vi "getDetails.vi"(8 "error in (no error)":errorcluster, 9 "S/N":string, 11 "reference in":refnum<class "Notification Controller.lvclass">) -> (0 "error out":errorcluster, 2 "details":T2, 3 "reference out":refnum<class "Notification Controller.lvclass">)   [LabVIEW 2014, in "Notification Controller.lvclass"]
uses:
  Notification Controller.lvclass
  Devices Controller_llb/deviceType.ctl
  APP/itemsNotification_class/itemsNotification.lvclass
  Devices Controller_llb/Devices Controller.lvclass
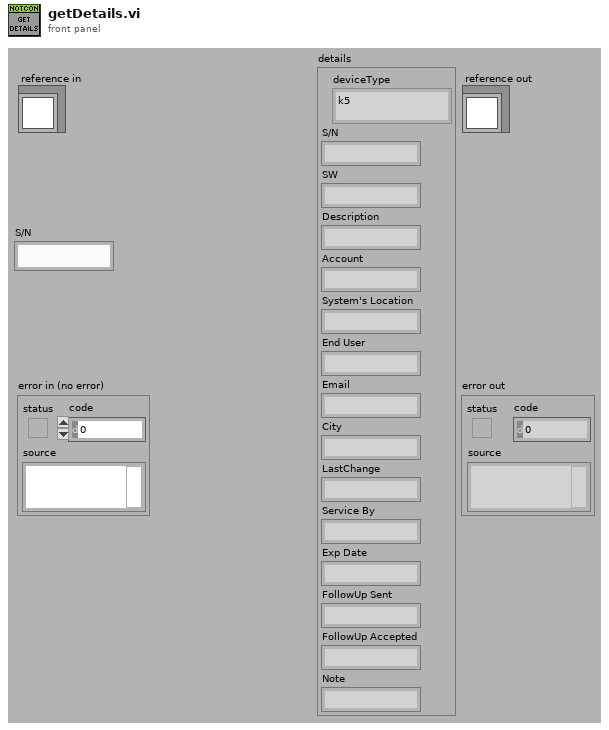
[diagram p1: front panel]
types:
  T1 = typedef "Devices Controller.lvclass/deviceType.ctl" = enum16{"k5", "k4b2", "fitmate", "cpet", "rmr", "bodyBoxPft", "bp", "pp"}
  T2 = cluster{"deviceType":T1, "S/N":string, "SW":string, "Description":string, "Account":string, "System's Location":string, "End User":string, "Email":string, "City":string, "LastChange":string, "Service By":string, "Exp Date":string, "FollowUp Sent":string, "FollowUp Accepted":string, "Note":string}
  T3 = typedef "Notification Controller.lvclass/ObjectAttributesRef.ctl" = refnum<data-value>
  T4 = typedef "Notification Controller.lvclass/ObjectAttributes.ctl" = cluster{"MyAttribute":dbl, "items_data":string[][][], "items_notification_refs":refnum<class "itemsNotification.lvclass">[], "notifications_data_items":string[][], "items_nots?":bool, "devices_controller_ref":refnum<class "Devices Controller.lvclass">, "onlineUpdate":timestamp, "notController?":bool, "tracking_notification_ref":refnum<class "trackingNotification.lvclass">, "notifications_data_tracking":string[][], "tracking_parts_data":string[][], "tracking_nots?":bool, "index_tracking_not":i32[], "file_controller_ref":refnum<class "File Controller.lvclass">}
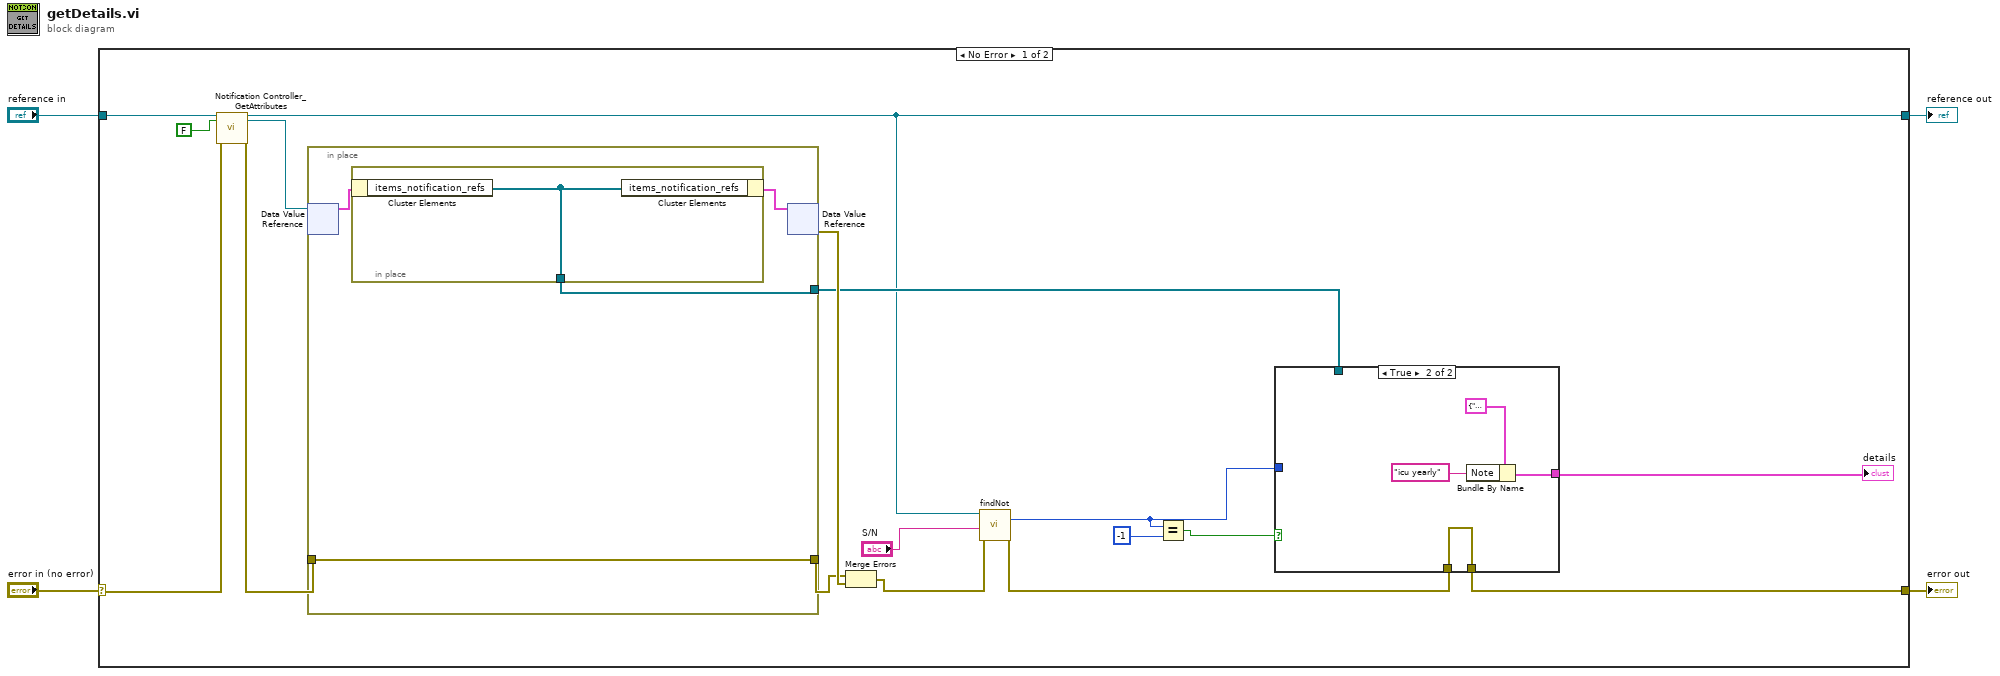
[diagram p0: block diagram]
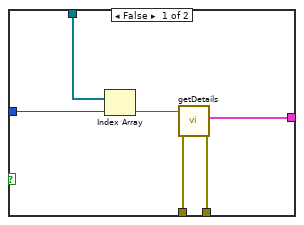
[diagram p2: hidden frame]
diagram:
  n1 = case shown="No Error" "error in (no error)" {
    selector: "error in (no error)" -> [w17 w38]
    tunnel: [w14 w38] -> w3
    tunnel: [w11 w37] -> w1
    tunnel: "reference in" -> [w19 w37]
    frame No Error {
      n2 = call "Notification Controller_GetAttributes.vi"("reference in"=w19, "return data? (T)"=FALSE, "error in (no error)"=w17) -> ("reference out"=w11:refnum<class "Notification Controller.lvclass">, "attributes ref"=w15:T3, "error out"=w16:errorcluster)  [unwired: 13 in, 1 out]
      n3 = in-place {
        in-place-border: w16 -> [w33]
        in-place-border: [w33] -> w20
        in-place-border: [w32] -> w12
        n4 = in-place-dvr #1(w15) -> (w34:T4)  [unwired: 1 out]
        n5 = in-place {
          in-place-border: [w36] -> w32
          n6 = in-place-cluster #2(w34) -> ("items_notification_refs"=w36:refnum<class "itemsNotification.lvclass">[])
          n7 = in-place-cluster #2("items_notification_refs"=w36) -> (w35:T4)
        }
        n8 = in-place-dvr #1(w35) -> (w21:errorcluster)  [unwired: 1 out]
      }
      n9 = Merge Errors(w20, w21) -> (w9:errorcluster)
      n10 = call "findNot.vi"("reference in"=w11, "S/N:"="S/N", "error in (no error)"=w9) -> ("index of element"=w7:i32, "error out"=w8:errorcluster)  [unwired: 13 in, 2 out]
      n11 = Equal?(x=w7, y=-1) -> (x = y?=w5:bool)
      n12 = case shown="True" w5 {
        tunnel: [w27 w31] -> w14
        tunnel: [w26 w29] -> w13
        tunnel: w12 -> [w25 _]
        tunnel: w8 -> [w24 w31]
        tunnel: w7 -> [w23 _]
        frame False {
          n13 = Index Array(array=w25, index=w23) -> (element=w22:refnum<class "itemsNotification.lvclass">)
          n14 = call "getDetails.vi"("error in (no error)"=w24, "reference in"=w22) -> ("error out"=w27:errorcluster, "details"=w26:T2)  [unwired: 7 in, 1 out]
        }
        frame True {
          n15 = Bundle By Name(cluster=T2 {"deviceType"=enum."k5", "S/N"="", "SW"="", "Description"="", "Account"="", "System's Location"="", "End User"="", "Email"="", "City"="", "LastChange"="", "Service By"="", "Exp Date"="", "FollowUp Sent"="", "FollowUp Accepted"="", "Note"=""} ("details 2"), "Note"="icu yearly") -> (w29:T2)
        }
      }
      "details" <- w13
    }
    frame Error {
    }
  }
  "error out" <- w3
  "reference out" <- w1
